vi "Run_Emergency_Stop.vi"(4 "error in (no error)":errorcluster) -> ()   [LabVIEW 2010]
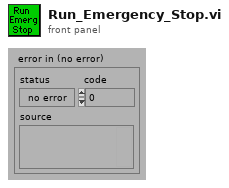
[diagram p1: front panel]
types:
  T1 = enum32{"Bad", "Idle", "Run top level", "Running"}
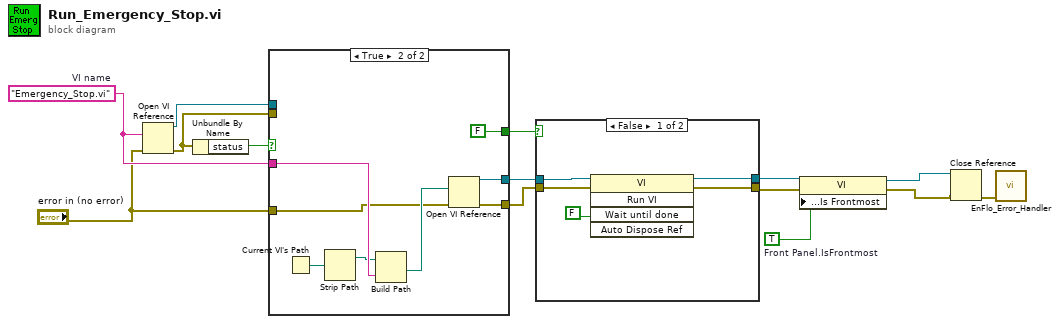
[diagram p0: block diagram]
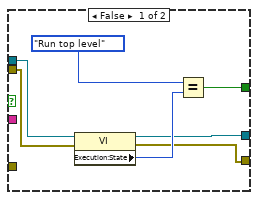
[diagram p3: hidden frame]
diagram:
  w1 = TRUE  # Front Panel.IsFrontmost
  w13 = "Emergency_Stop.vi"  # VI name
  n1 = Open VI Reference(vi path=w13, error in (no error)="error in (no error)") -> (vi reference=w11:refnum<vi>, error out=w12:errorcluster)  [unwired: 4 in]
  n2 = Unbundle By Name(w12) -> ("status"=w14:bool)
  n3 = case shown="True" w14 {
    tunnel: w13 -> [_ w28]
    tunnel: w12 -> [w21 _]
    tunnel: w11 -> [w20 _]
    tunnel: "error in (no error)" -> [_ w25]
    tunnel: [w17 FALSE] -> w8
    tunnel: [w16 w24] -> w7
    tunnel: [w15 w23] -> w6
    frame False {
      n4 = property class="VI"(reference=w20, error in=w21) -> (reference out=w16:refnum<vi>, error out=w15:errorcluster, "Execution:State"=w19:T1)
      n5 = Equal?(x=T1."Run top level" ("Exec.State"), y=w19) -> (x = y?=w17:bool)
    }
    frame True {
      n6 = Current VI's Path() -> (path=w29:path)
      n7 = Strip Path(path=w29) -> (stripped path=w27:path)  [unwired: 1 out]
      n8 = Build Path(base path=w27, name or relative path=w28) -> (appended path=w26:path)
      n9 = Open VI Reference(vi path=w26, error in (no error)=w25) -> (vi reference=w24:refnum<vi>, error out=w23:errorcluster)  [unwired: 4 in]
    }
  }
  n10 = case shown="False" w8 {
    tunnel: w7 -> [w32 w35]
    tunnel: w6 -> [w34 w36]
    tunnel: [w31 w36] -> w4
    tunnel: [w30 w35] -> w5
    frame False {
      n11 = invoke class="VI" method="Run VI"(reference=w32, error in=w34, "Wait until done"=FALSE) -> (reference out=w30:refnum<vi>, error out=w31:errorcluster)  [unwired: 2 in, 3 out]
    }
    frame True {
    }
  }
  n12 = property class="VI"(reference=w5, error in=w4, "Front Panel Window:Is Frontmost"=w1) -> (reference out=w2:refnum<vi>, error out=w3:errorcluster)
  n13 = Close Reference(reference=w2, error in (no error)=w3) -> (error out=w9:errorcluster)
  n14 = call "EnFlo_Error_Handler.vi"("error in (no error)"=w9) -> ()  [unwired: 2 in, 3 out]
